vi "Timestamp to string1.vi"(11 "time stamp":timestamp) -> (3 "string":string)   [LabVIEW 2017]
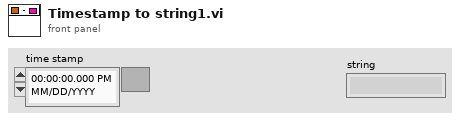
[diagram p1: front panel]
types:
  T1 = typedef "LVDateTimeRec.ctl" = cluster{"fractional second":dbl, "second":i32, "minute":i32, "hour":i32, "day of month":i32, "month":i32, "year":i32, "day of week":i32, "day of year":i32, "DST":i32}
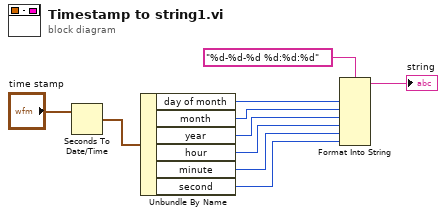
[diagram p0: block diagram]
diagram:
  n1 = Seconds To Date/Time(time stamp (now)="time stamp") -> (date time rec=w7:T1)  [unwired: 1 in]
  n2 = Unbundle By Name(w7) -> ("day of month"=w6:i32, "month"=w5:i32, "year"=w4:i32, "hour"=w3:i32, "minute"=w2:i32, "second"=w1:i32)
  n3 = Format Into String(format string="%d-%d-%d %d:%d:%d", w6, w5, w4, w3, w2, w1) -> (resulting string=→"string":string)  [unwired: 2 in, 1 out]
